vi "save_camera_signal_data.vi"(7 "Array of ROI sums":dbl[][][](array[numeric]), 8 "error in":errorcluster, 10 "XYZC iteration string":string, 11 "Data Files Path":path=path "C:/Users/QCC/Documents/Cesium_project/LabVIEW Projects/data/2011_03_02") -> (0 "error out":errorcluster)   [LabVIEW 2013]
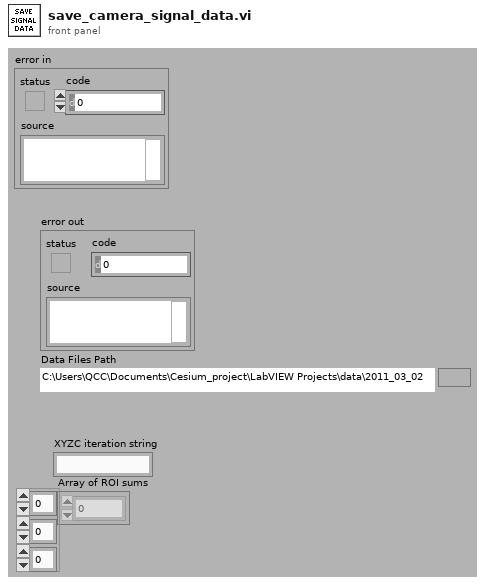
[diagram p1: front panel]
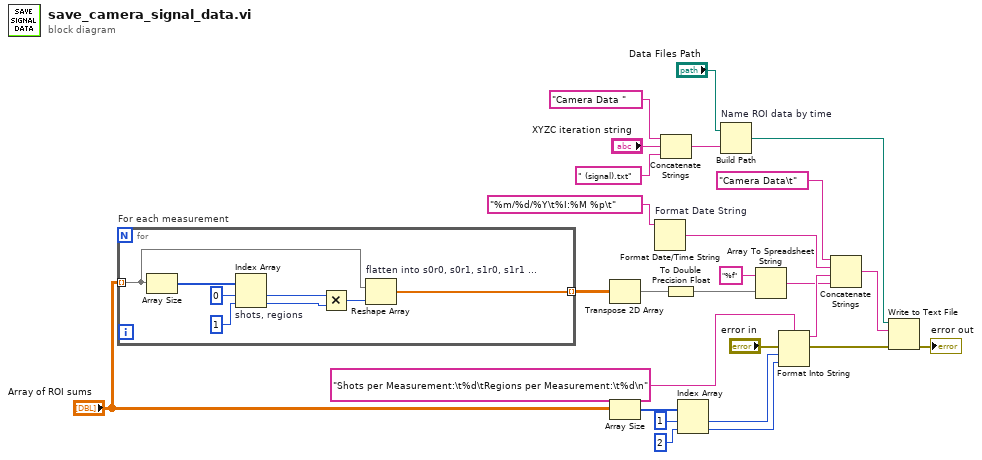
[diagram p0: block diagram]
diagram:
  n1 = for "For each measurement" {
    tunnel: "Array of ROI sums" -> [w34] mode=indexing
    tunnel: [w27] -> w1 mode=indexing
    n2 = Array Size(array=w34) -> (size(s)=w33:i32[])
    n3 = Index Array "shots, regions"(array=w33, index #1=0 ("index"), index #2=1 ("index")) -> (element #1=w30:i32, element #2=w29:i32)
    n4 = Multiply(x=w30, y=w29) -> (x*y=w28:i32)
    n5 = Reshape Array "flatten into s0r0, s0r1, s1r0, s1r1 ..."(w34, w28) -> (w27:dbl[])
  }
  n6 = Transpose 2D Array(2D array=w1) -> (transposed array=w16:dbl[][])
  n7 = Array Size(array="Array of ROI sums") -> (size(s)=w15:i32[])
  n8 = Format Date/Time String "Format Date String"(time format string (%c)="%m/%d/%Y\t%I:%M %p\t") -> (date/time string=w19:string)  [unwired: 2 in]
  n9 = Concatenate Strings("Camera Data ", "XYZC iteration string", " (signal).txt" ("string")) -> (w24:string)
  n10 = To Double Precision Float(number=w16) -> (double precision float=w3:dbl[][])
  n11 = Index Array(array=w15, index #1=1 ("index"), index #2=2 ("index")) -> (element #1=w5:i32, element #2=w4:i32)
  n12 = Build Path "Name ROI data by time"(base path="Data Files Path", name or relative path=w24) -> (appended path=w25:path)
  n13 = Array To Spreadsheet String(array=w3, 3:"%f" ("format string")) -> (spreadsheet string=w11:string)  [unwired: 1 in]
  n14 = Format Into String(format string="Shots per Measurement:\t%d\tRegions per Measurement:\t%d\n", error in="error in", w5, w4) -> (resulting string=w12:string, error out=w9:errorcluster)  [unwired: 1 in]
  n15 = Concatenate Strings("Camera Data\t", w19, w12, w11) -> (w18:string)
  n16 = Write to Text File(file (use dialog)=w25, text=w18, error in=w9) -> (error out=→"error out":errorcluster)  [unwired: 1 in, 2 out]
